vi "Histogram - NbRequirements Vs NbTestCases.vi"(8 "error in (no error)":errorcluster, 10 "XYGraph Ref":refnum<vi>, 11 "Pips in":refnum<class "Pips.lvclass">) -> (0 "error out":errorcluster, 1 "Image Data":T1, 2 "Nb Requirement with \"N\" Test Cases":cluster{i32[], i32[]}(graph), 3 "Pips out":refnum<class "Pips.lvclass">)   [LabVIEW 2021, in "Bananas.lvlib" / "Pips.lvclass"]
uses:
  Pips.lvclass
  pip_filter -- enum.ctl
  <vilib>/picture/picture.llb/imagedata.ctl
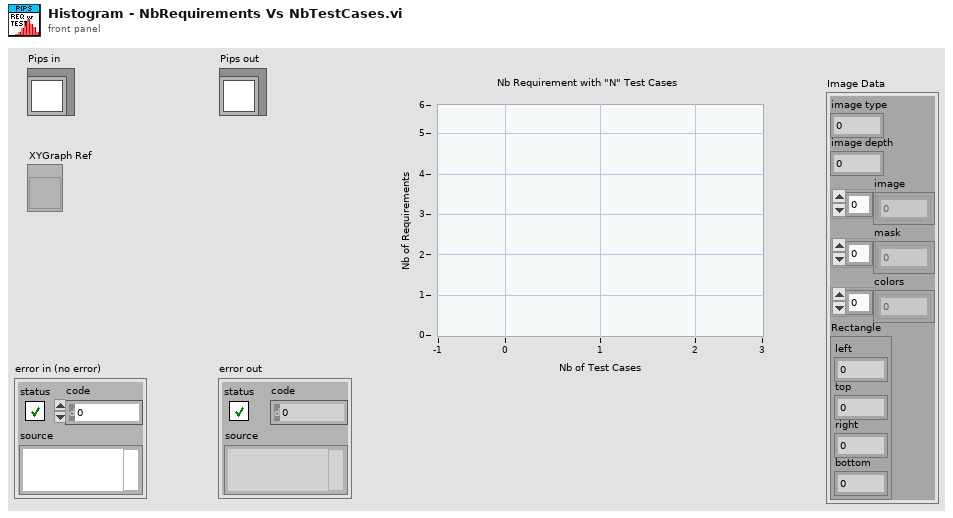
[diagram p1: front panel]
types:
  T1 = typedef "imagedata.ctl" = cluster{"image type":i32, "image depth":i32, "image":u8[], "mask":u8[], "colors":u32[], "Rectangle":cluster{"left":i16, "top":i16, "right":i16, "bottom":i16}}
  T2 = typedef "Bananas.lvlib/Pips.lvclass/pip_filter -- enum.ctl" = enum16{"none", "passed", "skipped", "failed", "blocked", "implemented", "covered", "uncovered", "partially-covered"}
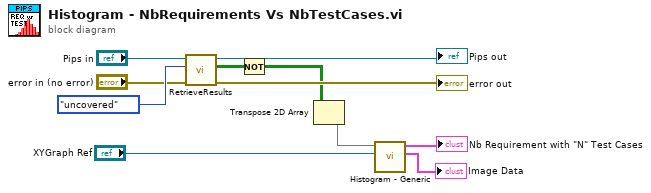
[diagram p0: block diagram]
diagram:
  n1 = call "RetrieveResults.vi"("error in (no error)"="error in (no error)", "Filter"=pip_filter_--_enum."uncovered", "Pips in"="Pips in") -> ("error out"=→"error out":errorcluster, "Matrix"=w10:bool[][], "Pips out"=→"Pips out":refnum<class "Pips.lvclass">)  [unwired: 6 in]
  n2 = Not(x=w10) -> (.not. x?=w2:bool[][])
  n3 = Transpose 2D Array(2D array=w2) -> (transposed array=w3:bool[][])
  n4 = call "Histogram - Generic.vi"("XYGraph Ref"="XYGraph Ref", "Matrix"=w3) -> ("Image Data"=→"Image Data":T1, "Nb of X per Y"=→"Nb Requirement with \"N\" Test Cases":cluster{i32[], i32[]})  [unwired: 8 in]
